vi "Thrust.vi"() -> ()   [LabVIEW 2018]
panel:
  out "Thurst Chart":dynamicdata(graph)
  in  "End Loop":bool
  out "?":dbl
  out "Thrust (Lbs)":dbl(knob) scale=0.0..2000.0
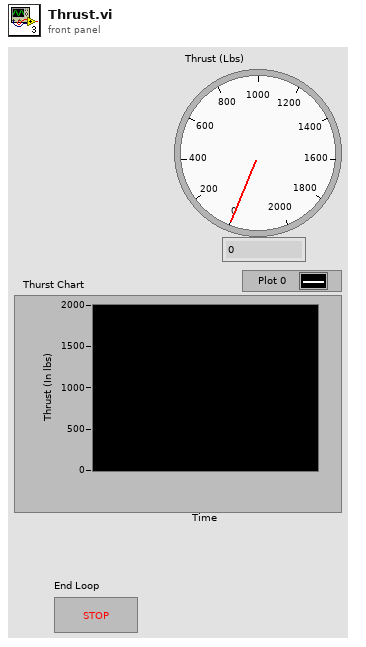
[diagram p1: front panel]
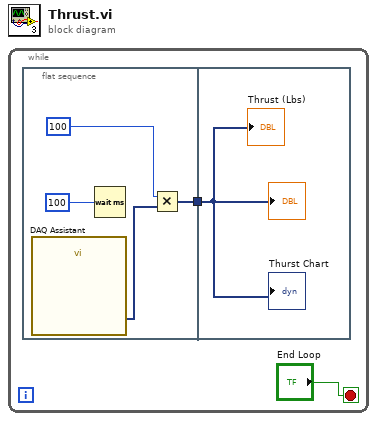
[diagram p0: block diagram]
diagram:
  n1 = while {
    stop <- "End Loop" stop-if-true
    n2 = flat-sequence {
      tunnel: [w5] -> w2
      tunnel: w2 -> [w7]
      frame #0 {
        n3 = call "DAQ Assistant"() -> ("data"=w3:dynamicdata)  [unwired: 17 in, 2 out]
        n4 = Wait (ms)(milliseconds to wait=100) -> ()  [unwired: 1 out]
        n5 = Multiply(x=100, y=w3) -> (x*y=w5:dynamicdata)
      }
      frame #1 {
        "Thrust (Lbs)" <- w7
        "?" <- w7
        "Thurst Chart" <- w7
      }
    }
  }
